vi "ControlsToClass.vi"(8 "ErrorArray":errorcluster[](array[cluster]), 11 "TestBase in":refnum<class "TestBase.lvclass">) -> (0 "ErrorArray":errorcluster[](array[cluster]), 3 "TestBase out":refnum<class "TestBase.lvclass">)   [LabVIEW 2014]
uses:
  TestBase.lvclass
  <userlib>/NIST/NISTErrorLib/NISTErrorLib.lvlib
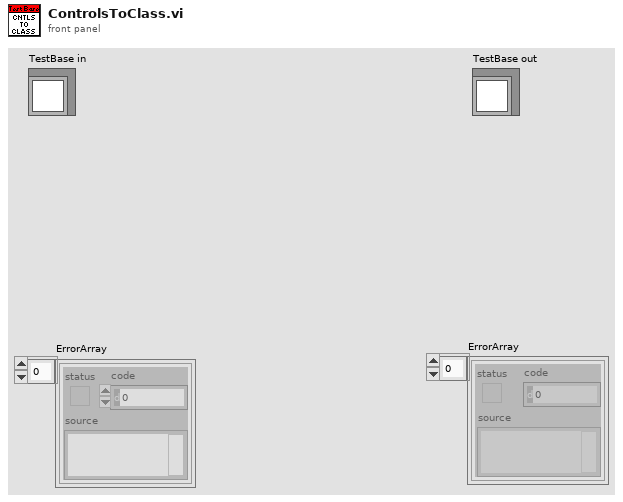
[diagram p1: front panel]
types:
  T1 = typedef "FpCntrlRefs.ctl" = cluster{"WfrmRingRef":refnum<vi>, "WfrmParams":refnum<vi>, "StartTime":refnum<vi>, "EndTime":refnum<vi>, "FGenRingRef":refnum<vi>, "SettleTime":refnum<vi>, "SyncRingRef":refnum<vi>, "SampRingRef":refnum<vi>, "AnalRingRef":refnum<vi>, "TstPathRef":refnum<vi>, "ScriptPathRef":refnum<vi>}
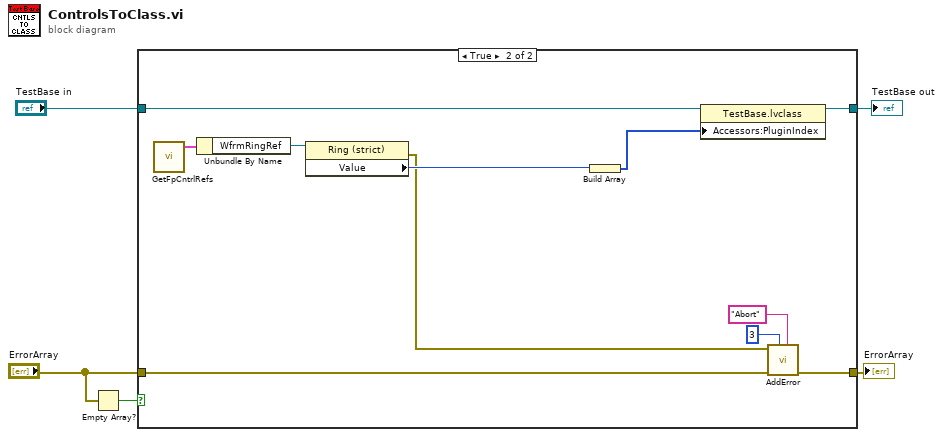
[diagram p0: block diagram]
diagram:
  n1 = Empty Array?(array="ErrorArray") -> (empty?=w2:bool)
  n2 = case shown="True" w2 {
    tunnel: [w7 w11] -> w1
    tunnel: [w6 w13] -> w4
    tunnel: "TestBase in" -> [w6 w18]
    tunnel: "ErrorArray" -> [w7 w17]
    frame False {
    }
    frame True {
      n3 = call "GetFpCntrlRefs.vi"() -> ("FpCntrlRefs"=w16:T1)  [unwired: 11 in]
      n4 = Unbundle By Name(w16) -> ("WfrmRingRef"=w15:refnum<vi>)
      n5 = property class="Ring (strict)"(reference=w15) -> (error out=w10:errorcluster, "Value"=w14:u16)  [unwired: 1 in, 1 out]
      n6 = Build Array(w14) -> (w12:u16[])
      n7 = property class="TestBase.lvclass"(reference=w18, "Accessors:PluginIndex"=w12) -> (reference out=w13:refnum<class "TestBase.lvclass">)  [unwired: 1 in, 1 out]
      n8 = call <userlib>:"AddError.vi"("Severity"="Abort", "Priority"=u8 3, "ErrorArray"=w17, "error in (no error)"=w10) -> ("ErrorArray"=w11:errorcluster[])  [unwired: 6 in, 1 out]
    }
  }
  "TestBase out" <- w4
  "ErrorArray" <- w1
